vi "Flush Data to Log File.vi"(8 "error in (no error)":errorcluster, 10 "Data Queue":refnum<queue>, 11 "Logging Configuration":T1) -> (0 "error out":errorcluster)   [LabVIEW 2013, in "Logging Logging.lvlib"]
doc: "Flush the data queue of any pending data and write it to the log file. Close the TDMS file reference."
uses:
  Logging Logging.lvlib
  Logging Configuration.ctl
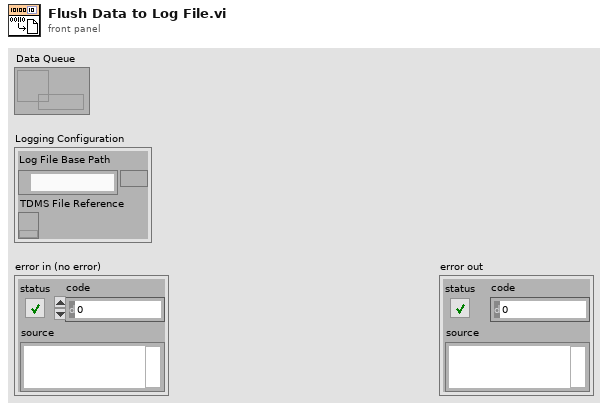
[diagram p1: front panel]
types:
  T1 = typedef "Logging Logging.lvlib/Logging Configuration.ctl" = cluster{"Log File Base Path":path, "TDMS File Reference":refnum<k34>}
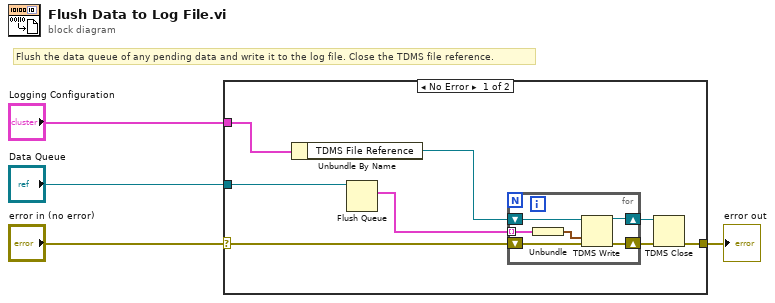
[diagram p0: block diagram]
diagram:
  # "Flush the data queue of any pending data and write it to the log file. Close the TDMS file reference."
  n1 = case shown="No Error" "error in (no error)" {
    selector: "error in (no error)" -> [w5 w19]
    tunnel: "Data Queue" -> [w8 _]
    tunnel: "Logging Configuration" -> [w7 _]
    tunnel: [w6 w19] -> w2
    frame No Error {
      n2 = Unbundle By Name(w7) -> ("TDMS File Reference"=w9:refnum<k34>)
      n3 = Flush Queue(queue=w8) -> (remaining elements=w12:cluster{"Array":waveform(dbl)[]}[])  [unwired: 1 in, 2 out]
      n4 = for {
        shift-right: [w15] -> w10
        shift-left: w9 -> [w16]
        shift-right: [w17] -> w11
        shift-left: w5 -> [w18]
        tunnel: w12 -> [w14] mode=indexing
        n5 = Unbundle(w14) -> ("Array"=w13:waveform(dbl)[])
        n6 = TDMS Write(0:w16, 9:w13, 11:w18) -> (4:w15:refnum<k34>, 15:w17:errorcluster)  [unwired: 3 in, 2 out]
      }
      n7 = TDMS Close(8:w11, 11:w10) -> (0:w6:errorcluster)  [unwired: 1 out]
    }
    frame Error {
    }
  }
  "error out" <- w2
